vi "Safely Disintegrate.vi"(11 "Bricks in":T1(array[cluster])) -> (3 "Number Disintegrated":i32)   [LabVIEW 2023, in "d22.lvlib"]
uses:
  d22.lvlib
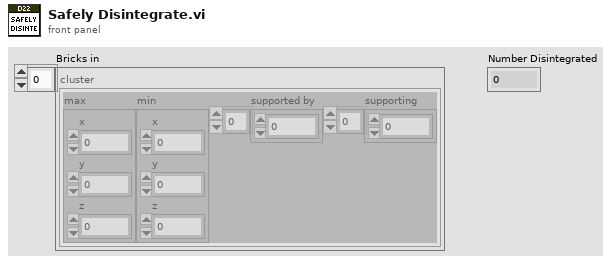
[diagram p1: front panel]
types:
  T1 = cluster{"max":cluster{"x":i32, "y":i32, "z":i32}, "min":cluster{"x":i32, "y":i32, "z":i32}, "supported by":i32[], "supporting":i32[]}[]
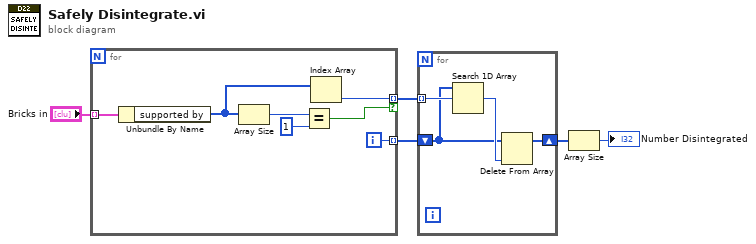
[diagram p0: block diagram]
diagram:
  n1 = for {
    tunnel: "Bricks in" -> [w12] mode=indexing
    tunnel: [w8] -> w3 mode=indexing if=w6
    tunnel: [w7] -> w2 mode=indexing
    i -> [w7]
    n2 = Unbundle By Name(w12) -> ("supported by"=w9:i32[])
    n3 = Array Size(array=w9) -> (size(s)=w11:i32)
    n4 = Equal?(x=w11, y=1) -> (x = y?=w6:bool)
    n5 = Index Array(array=w9) -> (element=w8:i32)  [unwired: 1 in]
  }
  n6 = for {
    tunnel: w3 -> [w16] mode=indexing
    shift-right: [w13] -> w4
    shift-left: w2 -> [w14]
    n7 = Search 1D Array(1D array=w14, element=w16) -> (index of element=w15:i32)  [unwired: 1 in]
    n8 = Delete From Array(array=w14, index=w15) -> (array with subset deleted=w13:i32[])  [unwired: 1 in, 1 out]
  }
  n9 = Array Size(array=w4) -> (size(s)=→"Number Disintegrated":i32)
